vi "Phase_unwrapping3.vi"() -> ()   [LabVIEW 2016]
panel:
  out "Array":dbl[](array[numeric])
  in  "Phase At Peaks":dbl[](array[numeric])=[0.0, 2.0, 3.0, 4.0]
  out "Array 3":dbl[](array[numeric])
  out "Missing Peaks":i32[](array[numeric])=[3, 4, 7, 8, 9]
  in  "Width":dbl=0.02 format="%#_13g"
  in  "Average Spacing":dbl=1.0 format="%#_13g"
  in  "Approximate Phase Difference":dbl=0.5 format="%#_13g"
  in  "Peak Locations":dbl[](array[numeric])=[0.0, 2.0, 3.0, 4.0]
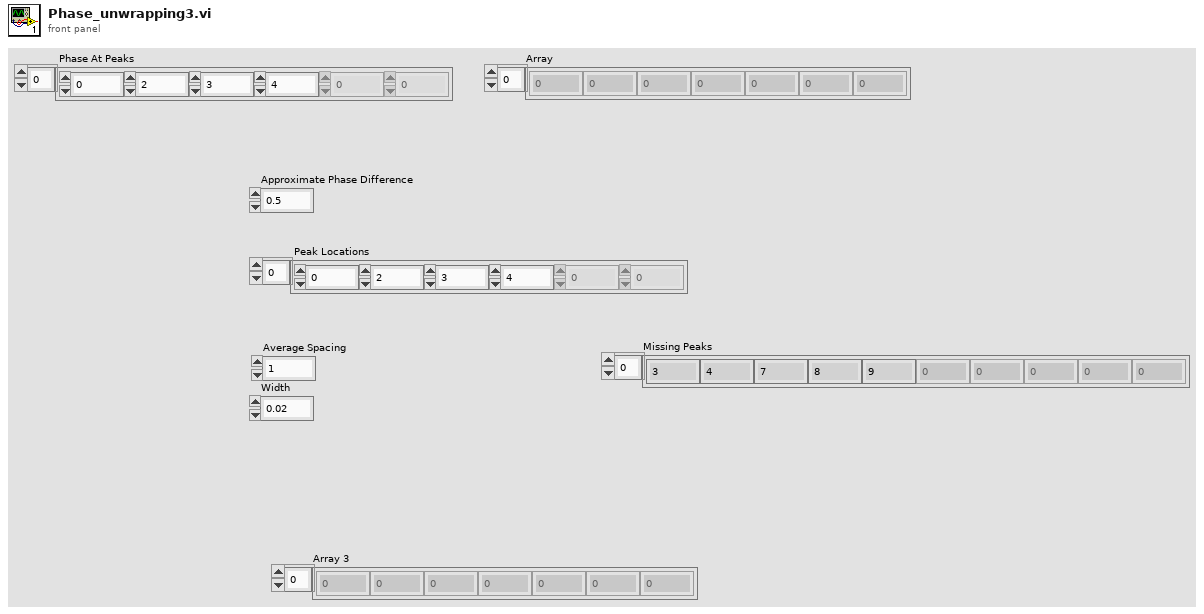
[diagram p1: front panel]
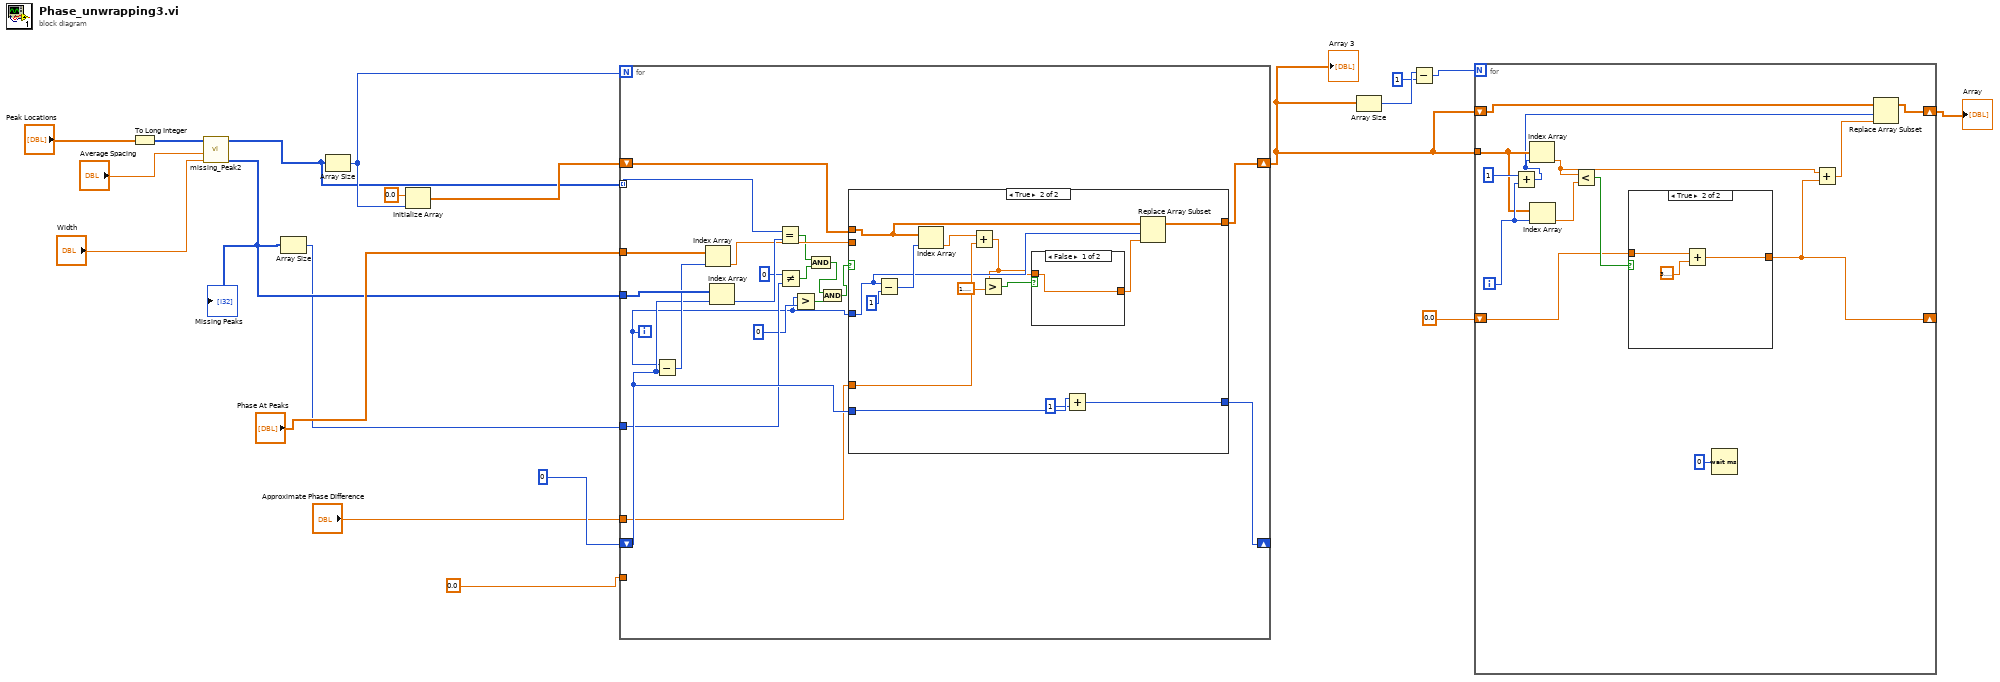
[diagram p0: block diagram]
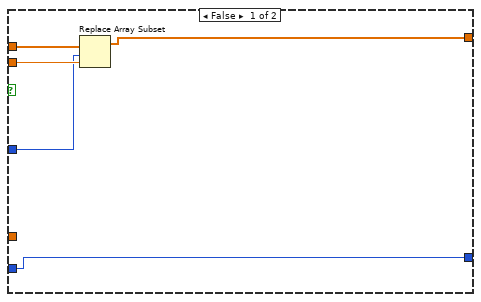
[diagram p3: hidden frame]
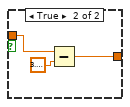
[diagram p4: hidden frame]
diagram:
  n1 = To Long Integer(number="Peak Locations") -> (32bit integer=w19:i32[])
  n2 = call "missing_Peak2.vi"("Width"="Width", "Average Spacing"="Average Spacing", 11:w19) -> ("Missing Peaks"=w10:i32[], "Padded Peak Locations"=w13:i32[])  [unwired: 7 in]
  "Missing Peaks" <- w10
  n3 = Array Size(array=w10) -> (size(s)=w9:i32)
  n4 = Array Size(array=w13) -> (size(s)=w15:i32)
  n5 = Initialize Array(0.0 ("element"), w15) -> (w14:dbl[])
  n6 = for {
    N: w15 -> [_]
    shift-right: [w21] -> w2
    shift-left: w14 -> [w36]
    tunnel: w13 -> [w37] mode=indexing
    shift-right: [w32] -> _
    shift-left: 0 -> [w33]
    tunnel: "Phase At Peaks" -> [w40]
    tunnel: w10 -> [w39]
    tunnel: w9 -> [w31]
    tunnel: "Approximate Phase Difference" -> [w27]
    tunnel: 0.0 -> [_]
    i -> [w22]
    n7 = Subtract(x=w22, y=w33) -> (x-y=w34:i32)
    n8 = Index Array(array=w40, index=w34) -> (element=w35:dbl)
    n9 = Index Array(array=w39, index=w33) -> (element=w38:i32)
    n10 = Equal?(x=w37, y=w38) -> (x = y?=w29:bool)
    n11 = Not Equal?(x=0, y=w31) -> (x != y?=w28:bool)
    n12 = Greater?(x=w22, y=0) -> (0:w24:bool)
    n13 = And(x=w29, y=w28) -> (x .and. y?=w26:bool)
    n14 = And(x=w26, y=w24) -> (x .and. y?=w25:bool)
    n15 = case shown="True" w25 {
      tunnel: w36 -> [w45 w52]
      tunnel: w35 -> [w44 _]
      tunnel: w22 -> [w43 w51]
      tunnel: [w42 w50] -> w21
      tunnel: w33 -> [w41 w59]
      tunnel: [w41 w57] -> w32
      tunnel: w27 -> [_ w53]
      frame False {
        n16 = Replace Array Subset(array=w45, new element=w44, index=w43) -> (w42:dbl[])
      }
      frame True {
        n17 = Subtract(x=w51, y=1) -> (x-y=w55:i32)
        n18 = Index Array(array=w52, index=w55) -> (element=w54:dbl)
        n19 = Add(x=w54, y=w53) -> (x+y=w47:dbl)
        n20 = Greater?(x=w47, y=1.5707963267948966) -> (0:w48:bool)
        n21 = case shown="False" w48 {
          tunnel: w47 -> [w60 w63]
          tunnel: [w60 w61] -> w46
          frame False {
          }
          frame True {
            n22 = Subtract(x=w63, y=3.141592653589793) -> (x-y=w61:dbl)
          }
        }
        n23 = Add(x=w59, y=1) -> (x+y=w57:i32)
        n24 = Replace Array Subset(array=w52, new element=w46, index=w51) -> (w50:dbl[])
      }
    }
  }
  "Array 3" <- w2
  n25 = Array Size(array=w2) -> (size(s)=w6:i32)
  n26 = Subtract(x=w6, y=1) -> (x-y=w5:i32)
  n27 = for {
    N: w5 -> [_]
    shift-right: [w64] -> _
    shift-left: 0.0 -> [w65]
    tunnel: w2 -> [w72]
    shift-right: [w67] -> w1
    shift-left: w2 -> [w68]
    i -> [w76]
    n28 = Add(x=1, y=w76) -> (x+y=w69:i32)
    n29 = Index Array(array=w72, index=w69) -> (element=w71:dbl)
    n30 = Index Array(array=w72, index=w76) -> (element=w74:dbl)
    n31 = Less?(x=w71, y=w74) -> (x < y?=w73:bool)
    n32 = case shown="True" w73 {
      tunnel: w65 -> [w77 w80]
      tunnel: [w77 w78] -> w64
      frame False {
      }
      frame True {
        n33 = Add(x=w80, y=3.141592653589793) -> (x+y=w78:dbl)
      }
    }
    n34 = Wait (ms)(milliseconds to wait=u32 0) -> ()  [unwired: 1 out]
    n35 = Add(x=w71, y=w64) -> (x+y=w70:dbl)
    n36 = Replace Array Subset(array=w68, new element=w70, index=w69) -> (w67:dbl[])
  }
  "Array" <- w1
